vi "Framework Test.vi"(6 "max iterations":u64=1000, 10 "channel values":dbl=13579.0 format="%.4f", 11 "channel selection":T1(ring)) -> (0 "error out":errorcluster, 3 "read = write":bool)   [LabVIEW 2021, in "Reentrancy Tests.lvclass"]
uses:
  Reentrancy Tests.lvclass
  Classes/Framework/Framework.lvclass
  <vilib>/NI/Memory Manager/Classes/Pointer/Pointer.lvclass
  Classes/Configuration Session/Configuration Session.lvclass
  Classes/Configuration/Core/Framework/Framework Configuration.lvclass
  <vilib>/NI/Memory Manager/Classes/Pointer/Write DBL.vi
  <vilib>/NI/Memory Manager/Classes/Pointer/Read DBL.vi
  Typedefs/DSF Engine Framework Configuration.ctl
  DSF Core.lvlib
  Classes/Framework/Framework Options.ctl
  Typedefs/DSF Performance Options.ctl
  Typedefs/DSF FIFO Options.ctl
  Classes/Thread/Thread Options.ctl
  Classes/Thread/Thread.lvclass
  Typedefs/DSF Plugin Options.ctl
  Classes/Framework/Data Server Options.ctl
  Typedefs/DSF Settings Info.ctl
  Typedefs/DSF Engine Plugin Thread Configuration.ctl
  Typedefs/DSF Engine Channel Configuration.ctl
  Typedefs/DSF Engine Transfer Configuration.ctl
  Typedefs/DSF Engine Transfer Group Configuration.ctl
  Typedefs/DSF Engine Plugin Configuration.ctl
  Typedefs/DSF Timing Info.ctl
  Typedefs/Core Plugin Configuration.ctl
  Classes/Configuration/Core/Plugin/Plugin Configuration.lvclass
  Typedefs/Core Thread Configuration.ctl
  Classes/Configuration/Core/Thread/Thread Configuration.lvclass
  Typedefs/DSF Direction.ctl
  Typedefs/DSF Timeout Behavior.ctl
  Typedefs/Core Group Configuration.ctl
  Classes/Configuration/Core/Group/Group Configuration.lvclass
  Typedefs/Core Transfer Configuration.ctl
  Classes/Configuration/Core/Transfer/Transfer Configuration.lvclass
  Typedefs/DSF Data Type.ctl
  Typedefs/Core Channel Configuration.ctl
  Classes/Configuration/Core/Channel/Channel Configuration.lvclass
panel:
  out "iteration":u64
  in  "framework options":T2={"FIFO Options"={"Infinite Timeouts"=FALSE}, "Thread Options"={"Show FP On Call"=TRUE, "Close FP After Call"=TRUE, "Allow Debugging"=TRUE}, "Plugin Options"={"Default Components"=TRUE}, "Performance Options"={"Measure Period"=TRUE, "Measure Rx/Tx Duration"=TRUE}, "Data Server Options"={"Enable Data Server"=TRUE, "Period"=50}} {"Data Server Options"."Period" format="%d ms"}
  in  "framework configuration":T8={"plugins"=[{"core"={"name"="Plugin", "components"=[], "cycle timing"={"priority"=10000, "decimation"=1, "offset"=0}}, "component settings"=[], "threads"=[{"core"={"processor"=-2, "priority offset"=0}, "component settings"=[], "transfer groups"=[{"core"={"name"="Group", "direction"=enum."Tx", "cycle timing"={"priority"=100, "decimation"=1, "offset"=0}, "timeout behavior"=enum."Increment Late Count", "enable conversion"=FALSE}, "component settings"=[], "transfers"=[{"core"={"name"="Transfer"}, "component settings"=[], "channels"=[{"core"={"name"="Channel", "units"="V", "engine data type"=enum."DBL", "string data type"=enum."DBL", "string offset"=0}, "component settings"=[]}, {"core"={"name"="Channel", "units"="V", "engine data type"=enum."DBL", "string data type"=enum."DBL", "string offset"=0}, "component settings"=[]}, {"core"={"name"="Channel", "units"="V", "engine data type"=enum."DBL", "string data type"=enum."DBL", "string offset"=0}, "component settings"=[]}, {"core"={"name"="Channel", "units"="V", "engine data type"=enum."DBL", "string data type"=enum."DBL", "string offset"=0}, "component settings"=[]}, {"core"={"name"="Channel", "units"="V", "engine data type"=enum."DBL", "string data type"=enum."DBL", "string offset"=0}, "component settings"=[]}, {"core"={"name"="Channel", "units"="V", "engine data type"=enum."DBL", "string data type"=enum."DBL", "string offset"=0}, "component settings"=[]}, {"core"={"name"="Channel", "units"="V", "engine data type"=enum."DBL", "string data type"=enum."DBL", "string offset"=0}, "component settings"=[]}, {"core"={"name"="Channel", "units"="V", "engine data type"=enum."DBL", "string data type"=enum."DBL", "string offset"=0}, "component settings"=[]}, {"core"={"name"="Channel", "units"="V", "engine data type"=enum."DBL", "string data type"=enum."DBL", "string offset"=0}, "component settings"=[]}, {"core"={"name"="Channel", "units"="V", "engine data type"=enum."DBL", "string data type"=enum."DBL", "string offset"=0}, "component settings"=[]}, {"core"={"name"="Channel", "units"="V", "engine data type"=enum."DBL", "string data type"=enum."DBL", "string offset"=0}, "component settings"=[]}, {"core"={"name"="Channel", "units"="V", "engine data type"=enum."DBL", "string data type"=enum."DBL", "string offset"=0}, "component settings"=[]}, {"core"={"name"="Channel", "units"="V", "engine data type"=enum."DBL", "string data type"=enum."DBL", "string offset"=0}, "component settings"=[]}, {"core"={"name"="Channel", "units"="V", "engine data type"=enum."DBL", "string data type"=enum."DBL", "string offset"=0}, "component settings"=[]}, {"core"={"name"="Channel", "units"="V", "engine data type"=enum."DBL", "string data type"=enum."DBL", "string offset"=0}, "component settings"=[]}, {"core"={"name"="Channel", "units"="V", "engine data type"=enum."DBL", "string data type"=enum."DBL", "string offset"=0}, "component settings"=[]}, {"core"={"name"="Channel", "units"="V", "engine data type"=enum."DBL", "string data type"=enum."DBL", "string offset"=0}, "component settings"=[]}, {"core"={"name"="Channel", "units"="V", "engine data type"=enum."DBL", "string data type"=enum."DBL", "string offset"=0}, "component settings"=[]}, {"core"={"name"="Channel", "units"="V", "engine data type"=enum."DBL", "string data type"=enum."DBL", "string offset"=0}, "component settings"=[]}, {"core"={"name"="Channel", "units"="V", "engine data type"=enum."DBL", "string data type"=enum."DBL", "string offset"=0}, "component settings"=[]}, {"core"={"name"="Channel", "units"="V", "engine data type"=enum."DBL", "string data type"=enum."DBL", "string offset"=0}, "component settings"=[]}, {"core"={"name"="Channel", "units"="V", "engine data type"=enum."DBL", "string data type"=enum."DBL", "string offset"=0}, "component settings"=[]}, {"core"={"name"="Channel", "units"="V", "engine data type"=enum."DBL", "string data type"=enum."DBL", "string offset"=0}, "component settings"=[]}, {"core"={"name"="Channel", "units"="V", "engine data type"=enum."DBL", "string data type"=enum."DBL", "string offset"=0}, "component settings"=[]}, {"core"={"name"="Channel", "units"="V", "engine data type"=enum."DBL", "string data type"=enum."DBL", "string offset"=0}, "component settings"=[]}, {"core"={"name"="Channel", "units"="V", "engine data type"=enum."DBL", "string data type"=enum."DBL", "string offset"=0}, "component settings"=[]}, {"core"={"name"="Channel", "units"="V", "engine data type"=enum."DBL", "string data type"=enum."DBL", "string offset"=0}, "component settings"=[]}, {"core"={"name"="Channel", "units"="V", "engine data type"=enum."DBL", "string data type"=enum."DBL", "string offset"=0}, "component settings"=[]}, {"core"={"name"="Channel", "units"="V", "engine data type"=enum."DBL", "string data type"=enum."DBL", "string offset"=0}, "component settings"=[]}, {"core"={"name"="Channel", "units"="V", "engine data type"=enum."DBL", "string data type"=enum."DBL", "string offset"=0}, "component settings"=[]}, {"core"={"name"="Channel", "units"="V", "engine data type"=enum."DBL", "string data type"=enum."DBL", "string offset"=0}, "component settings"=[]}, {"core"={"name"="Channel", "units"="V", "engine data type"=enum."DBL", "string data type"=enum."DBL", "string offset"=0}, "component settings"=[]}, {"core"={"name"="Channel", "units"="V", "engine data type"=enum."DBL", "string data type"=enum."DBL", "string offset"=0}, "component settings"=[]}, {"core"={"name"="Channel", "units"="V", "engine data type"=enum."DBL", "string data type"=enum."DBL", "string offset"=0}, "component settings"=[]}, {"core"={"name"="Channel", "units"="V", "engine data type"=enum."DBL", "string data type"=enum."DBL", "string offset"=0}, "component settings"=[]}, {"core"={"name"="Channel", "units"="V", "engine data type"=enum."DBL", "string data type"=enum."DBL", "string offset"=0}, "component settings"=[]}, {"core"={"name"="Channel", "units"="V", "engine data type"=enum."DBL", "string data type"=enum."DBL", "string offset"=0}, "component settings"=[]}, {"core"={"name"="Channel", "units"="V", "engine data type"=enum."DBL", "string data type"=enum."DBL", "string offset"=0}, "component settings"=[]}, {"core"={"name"="Channel", "units"="V", "engine data type"=enum."DBL", "string data type"=enum."DBL", "string offset"=0}, "component settings"=[]}, {"core"={"name"="Channel", "units"="V", "engine data type"=enum."DBL", "string data type"=enum."DBL", "string offset"=0}, "component settings"=[]}, {"core"={"name"="Channel", "units"="V", "engine data type"=enum."DBL", "string data type"=enum."DBL", "string offset"=0}, "component settings"=[]}, {"core"={"name"="Channel", "units"="V", "engine data type"=enum."DBL", "string data type"=enum."DBL", "string offset"=0}, "component settings"=[]}, {"core"={"name"="Channel", "units"="V", "engine data type"=enum."DBL", "string data type"=enum."DBL", "string offset"=0}, "component settings"=[]}, {"core"={"name"="Channel", "units"="V", "engine data type"=enum."DBL", "string data type"=enum."DBL", "string offset"=0}, "component settings"=[]}, {"core"={"name"="Channel", "units"="V", "engine data type"=enum."DBL", "string data type"=enum."DBL", "string offset"=0}, "component settings"=[]}, {"core"={"name"="Channel", "units"="V", "engine data type"=enum."DBL", "string data type"=enum."DBL", "string offset"=0}, "component settings"=[]}, {"core"={"name"="Channel", "units"="V", "engine data type"=enum."DBL", "string data type"=enum."DBL", "string offset"=0}, "component settings"=[]}, {"core"={"name"="Channel", "units"="V", "engine data type"=enum."DBL", "string data type"=enum."DBL", "string offset"=0}, "component settings"=[]}, {"core"={"name"="Channel", "units"="V", "engine data type"=enum."DBL", "string data type"=enum."DBL", "string offset"=0}, "component settings"=[]}, {"core"={"name"="Channel", "units"="V", "engine data type"=enum."DBL", "string data type"=enum."DBL", "string offset"=0}, "component settings"=[]}, {"core"={"name"="Channel", "units"="V", "engine data type"=enum."DBL", "string data type"=enum."DBL", "string offset"=0}, "component settings"=[]}, {"core"={"name"="Channel", "units"="V", "engine data type"=enum."DBL", "string data type"=enum."DBL", "string offset"=0}, "component settings"=[]}, {"core"={"name"="Channel", "units"="V", "engine data type"=enum."DBL", "string data type"=enum."DBL", "string offset"=0}, "component settings"=[]}, {"core"={"name"="Channel", "units"="V", "engine data type"=enum."DBL", "string data type"=enum."DBL", "string offset"=0}, "component settings"=[]}, {"core"={"name"="Channel", "units"="V", "engine data type"=enum."DBL", "string data type"=enum."DBL", "string offset"=0}, "component settings"=[]}, {"core"={"name"="Channel", "units"="V", "engine data type"=enum."DBL", "string data type"=enum."DBL", "string offset"=0}, "component settings"=[]}, {"core"={"name"="Channel", "units"="V", "engine data type"=enum."DBL", "string data type"=enum."DBL", "string offset"=0}, "component settings"=[]}, {"core"={"name"="Channel", "units"="V", "engine data type"=enum."DBL", "string data type"=enum."DBL", "string offset"=0}, "component settings"=[]}, {"core"={"name"="Channel", "units"="V", "engine data type"=enum."DBL", "string data type"=enum."DBL", "string offset"=0}, "component settings"=[]}, {"core"={"name"="Channel", "units"="V", "engine data type"=enum."DBL", "string data type"=enum."DBL", "string offset"=0}, "component settings"=[]}, {"core"={"name"="Channel", "units"="V", "engine data type"=enum."DBL", "string data type"=enum."DBL", "string offset"=0}, "component settings"=[]}, {"core"={"name"="Channel", "units"="V", "engine data type"=enum."DBL", "string data type"=enum."DBL", "string offset"=0}, "component settings"=[]}, {"core"={"name"="Channel", "units"="V", "engine data type"=enum."DBL", "string data type"=enum."DBL", "string offset"=0}, "component settings"=[]}, {"core"={"name"="Channel", "units"="V", "engine data type"=enum."DBL", "string data type"=enum."DBL", "string offset"=0}, "component settings"=[]}, {"core"={"name"="Channel", "units"="V", "engine data type"=enum."DBL", "string data type"=enum."DBL", "string offset"=0}, "component settings"=[]}, {"core"={"name"="Channel", "units"="V", "engine data type"=enum."DBL", "string data type"=enum."DBL", "string offset"=0}, "component settings"=[]}, {"core"={"name"="Channel", "units"="V", "engine data type"=enum."DBL", "string data type"=enum."DBL", "string offset"=0}, "component settings"=[]}, {"core"={"name"="Channel", "units"="V", "engine data type"=enum."DBL", "string data type"=enum."DBL", "string offset"=0}, "component settings"=[]}, {"core"={"name"="Channel", "units"="V", "engine data type"=enum."DBL", "string data type"=enum."DBL", "string offset"=0}, "component settings"=[]}, {"core"={"name"="Channel", "units"="V", "engine data type"=enum."DBL", "string data type"=enum."DBL", "string offset"=0}, "component settings"=[]}, {"core"={"name"="Channel", "units"="V", "engine data type"=enum."DBL", "string data type"=enum."DBL", "string offset"=0}, "component settings"=[]}, {"core"={"name"="Channel", "units"="V", "engine data type"=enum."DBL", "string data type"=enum."DBL", "string offset"=0}, "component settings"=[]}, {"core"={"name"="Channel", "units"="V", "engine data type"=enum."DBL", "string data type"=enum."DBL", "string offset"=0}, "component settings"=[]}, {"core"={"name"="Channel", "units"="V", "engine data type"=enum."DBL", "string data type"=enum."DBL", "string offset"=0}, "component settings"=[]}, {"core"={"name"="Channel", "units"="V", "engine data type"=enum."DBL", "string data type"=enum."DBL", "string offset"=0}, "component settings"=[]}, {"core"={"name"="Channel", "units"="V", "engine data type"=enum."DBL", "string data type"=enum."DBL", "string offset"=0}, "component settings"=[]}, {"core"={"name"="Channel", "units"="V", "engine data type"=enum."DBL", "string data type"=enum."DBL", "string offset"=0}, "component settings"=[]}, {"core"={"name"="Channel", "units"="V", "engine data type"=enum."DBL", "string data type"=enum."DBL", "string offset"=0}, "component settings"=[]}, {"core"={"name"="Channel", "units"="V", "engine data type"=enum."DBL", "string data type"=enum."DBL", "string offset"=0}, "component settings"=[]}, {"core"={"name"="Channel", "units"="V", "engine data type"=enum."DBL", "string data type"=enum."DBL", "string offset"=0}, "component settings"=[]}, {"core"={"name"="Channel", "units"="V", "engine data type"=enum."DBL", "string data type"=enum."DBL", "string offset"=0}, "component settings"=[]}, {"core"={"name"="Channel", "units"="V", "engine data type"=enum."DBL", "string data type"=enum."DBL", "string offset"=0}, "component settings"=[]}, {"core"={"name"="Channel", "units"="V", "engine data type"=enum."DBL", "string data type"=enum."DBL", "string offset"=0}, "component settings"=[]}, {"core"={"name"="Channel", "units"="V", "engine data type"=enum."DBL", "string data type"=enum."DBL", "string offset"=0}, "component settings"=[]}, {"core"={"name"="Channel", "units"="V", "engine data type"=enum."DBL", "string data type"=enum."DBL", "string offset"=0}, "component settings"=[]}, {"core"={"name"="Channel", "units"="V", "engine data type"=enum."DBL", "string data type"=enum."DBL", "string offset"=0}, "component settings"=[]}, {"core"={"name"="Channel", "units"="V", "engine data type"=enum."DBL", "string data type"=enum."DBL", "string offset"=0}, "component settings"=[]}, {"core"={"name"="Channel", "units"="V", "engine data type"=enum."DBL", "string data type"=enum."DBL", "string offset"=0}, "component settings"=[]}, {"core"={"name"="Channel", "units"="V", "engine data type"=enum."DBL", "string data type"=enum."DBL", "string offset"=0}, "component settings"=[]}, {"core"={"name"="Channel", "units"="V", "engine data type"=enum."DBL", "string data type"=enum."DBL", "string offset"=0}, "component settings"=[]}, {"core"={"name"="Channel", "units"="V", "engine data type"=enum."DBL", "string data type"=enum."DBL", "string offset"=0}, "component settings"=[]}, {"core"={"name"="Channel", "units"="V", "engine data type"=enum."DBL", "string data type"=enum."DBL", "string offset"=0}, "component settings"=[]}, {"core"={"name"="Channel", "units"="V", "engine data type"=enum."DBL", "string data type"=enum."DBL", "string offset"=0}, "component settings"=[]}, {"core"={"name"="Channel", "units"="V", "engine data type"=enum."DBL", "string data type"=enum."DBL", "string offset"=0}, "component settings"=[]}, {"core"={"name"="Channel", "units"="V", "engine data type"=enum."DBL", "string data type"=enum."DBL", "string offset"=0}, "component settings"=[]}, {"core"={"name"="Channel", "units"="V", "engine data type"=enum."DBL", "string data type"=enum."DBL", "string offset"=0}, "component settings"=[]}, {"core"={"name"="Channel", "units"="V", "engine data type"=enum."DBL", "string data type"=enum."DBL", "string offset"=0}, "component settings"=[]}, {"core"={"name"="Channel", "units"="V", "engine data type"=enum."DBL", "string data type"=enum."DBL", "string offset"=0}, "component settings"=[]}, {"core"={"name"="Channel", "units"="V", "engine data type"=enum."DBL", "string data type"=enum."DBL", "string offset"=0}, "component settings"=[]}, {"core"={"name"="Channel", "units"="V", "engine data type"=enum."DBL", "string data type"=enum."DBL", "string offset"=0}, "component settings"=[]}]}]}]}]}]}
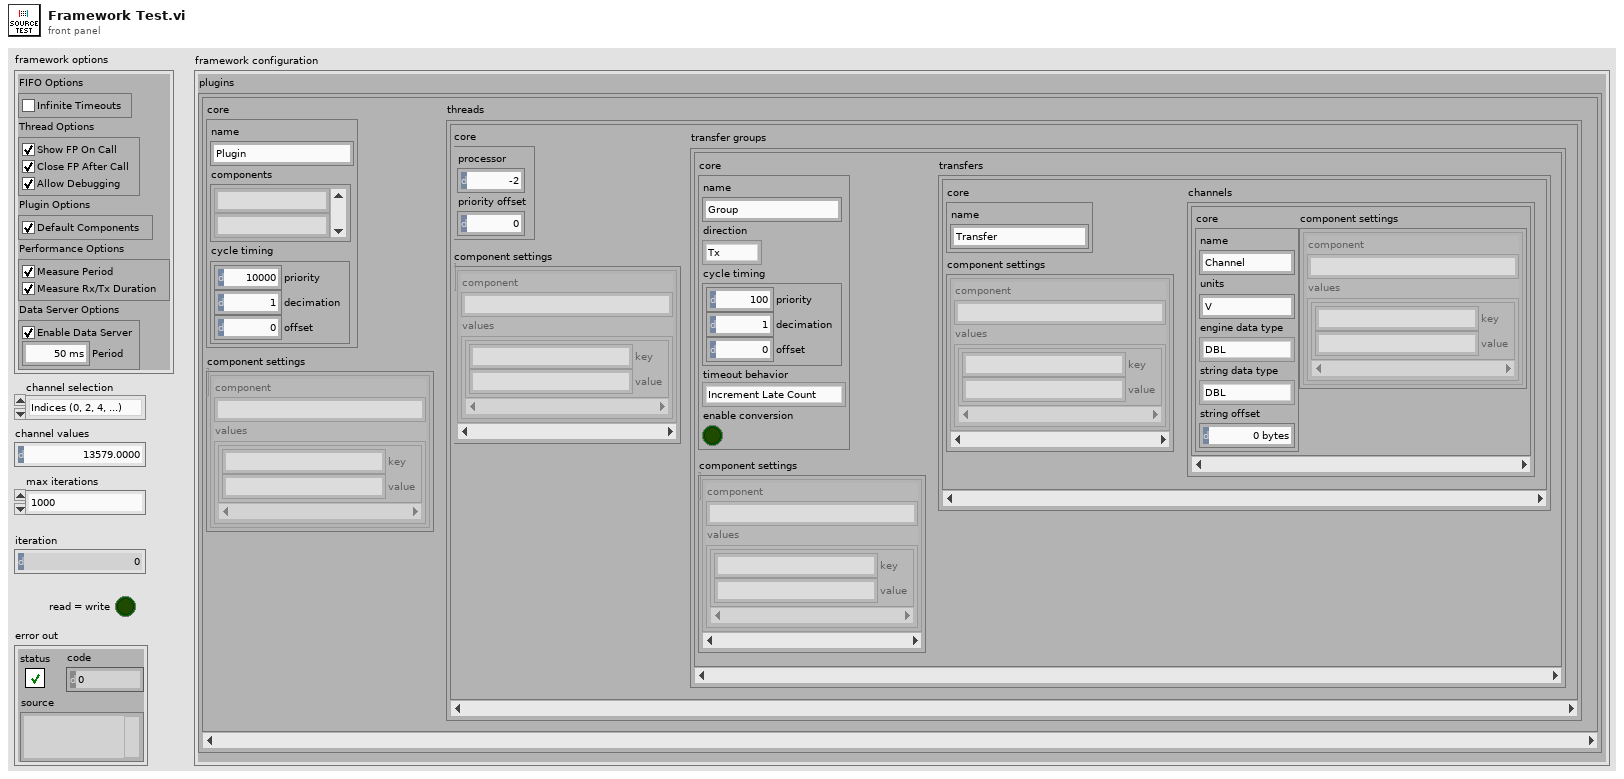
[diagram p1: front panel]
types:
  T1 = enum16{"Indices (0, 2, 4, ...)", "Indices (1, 3, 5, ...)", "All"}
  T2 = typedef "DSF Core.lvlib/Framework.lvclass/Framework Options.ctl" = cluster{"FIFO Options":T3, "Thread Options":T4, "Plugin Options":T5, "Performance Options":T6, "Data Server Options":T7}
  T3 = typedef "DSF Core.lvlib/Framework.lvclass/DSF FIFO Options.ctl" = cluster{"Infinite Timeouts":bool}
  T4 = typedef "DSF Core.lvlib/Thread.lvclass/Thread Options.ctl" = cluster{"Show FP On Call":bool, "Close FP After Call":bool, "Allow Debugging":bool}
  T5 = typedef "DSF Core.lvlib/Framework.lvclass/DSF Plugin Options.ctl" = cluster{"Default Components":bool}
  T6 = typedef "DSF Core.lvlib/DSF Performance Options.ctl" = cluster{"Measure Period":bool, "Measure Rx/Tx Duration":bool}
  T7 = typedef "DSF Core.lvlib/Framework.lvclass/Data Server Options.ctl" = cluster{"Enable Data Server":bool, "Period":u32}
  T8 = typedef "DSF Core.lvlib/DSF Engine Framework Configuration.ctl" = cluster{"plugins":T9[]}
  T9 = typedef "DSF Core.lvlib/DSF Engine Plugin Configuration.ctl" = cluster{"core":T10, "component settings":T12[], "threads":T13[]}
  T10 = typedef "DSF Core.lvlib/Plugin Configuration.lvclass/Core Plugin Configuration.ctl" = cluster{"name":string, "components":string[], "cycle timing":T11}
  T11 = typedef "DSF Core.lvlib/DSF Timing Info.ctl" = cluster{"priority":u64, "decimation":u64, "offset":u64}
  T12 = typedef "DSF Core.lvlib/DSF Settings Info.ctl" = cluster{"component":string, "values":cluster{"key":string, "value":string}[]}
  T13 = typedef "DSF Core.lvlib/DSF Engine Plugin Thread Configuration.ctl" = cluster{"core":T14, "component settings":T12[], "transfer groups":T15[]}
  T14 = typedef "DSF Core.lvlib/Thread Configuration.lvclass/Core Thread Configuration.ctl" = cluster{"processor":i32, "priority offset":i16}
  T15 = typedef "DSF Core.lvlib/DSF Engine Transfer Group Configuration.ctl" = cluster{"core":T16, "component settings":T12[], "transfers":T19[]}
  T16 = typedef "DSF Core.lvlib/Group Configuration.lvclass/Core Group Configuration.ctl" = cluster{"name":string, "direction":T17, "cycle timing":T11, "timeout behavior":T18, "enable conversion":bool}
  T17 = typedef "DSF Core.lvlib/DSF Direction.ctl" = enum8{"Tx", "Rx"}
  T18 = typedef "DSF Core.lvlib/DSF Timeout Behavior.ctl" = enum8{"Increment Late Count", "Throw Error"}
  T19 = typedef "DSF Core.lvlib/DSF Engine Transfer Configuration.ctl" = cluster{"core":T20, "component settings":T12[], "channels":T21[]}
  T20 = typedef "DSF Core.lvlib/Transfer Configuration.lvclass/Core Transfer Configuration.ctl" = cluster{"name":string}
  T21 = typedef "DSF Core.lvlib/DSF Engine Channel Configuration.ctl" = cluster{"core":T22, "component settings":T12[]}
  T22 = typedef "DSF Core.lvlib/Channel Configuration.lvclass/Core Channel Configuration.ctl" = cluster{"name":string, "units":string, "engine data type":T23, "string data type":T23, "string offset":u64}
  T23 = typedef "DSF Core.lvlib/DSF Data Type.ctl" = enum8{"Bool", "SGL", "DBL", "I8", "I16", "I32", "I64", "U8", "U16", "U32", "U64"}
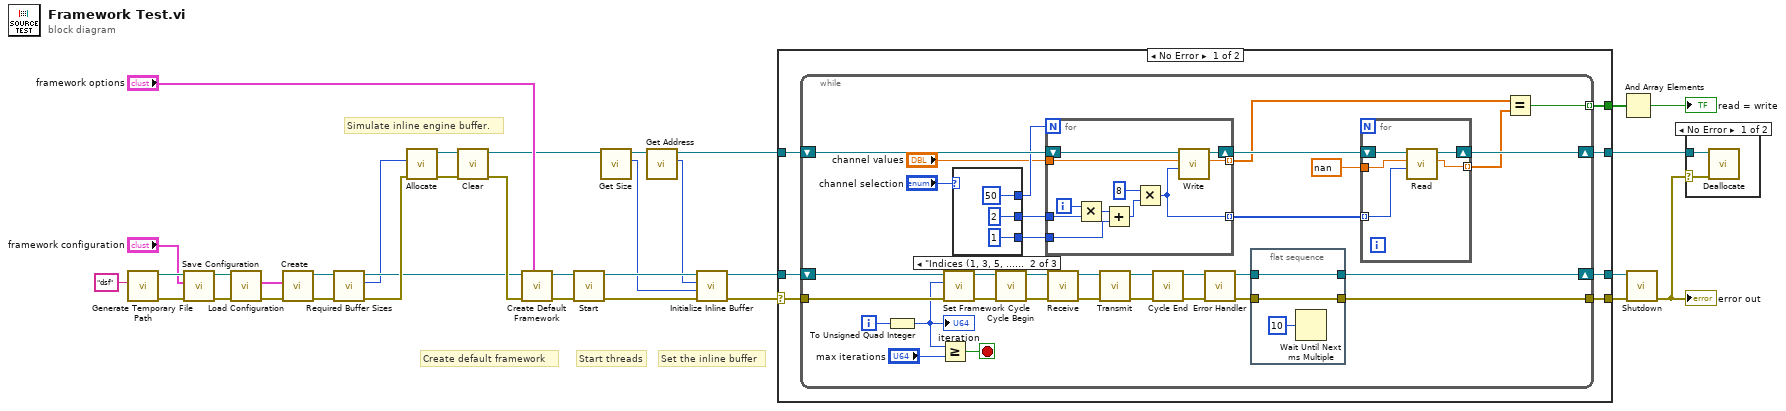
[diagram p0: block diagram]
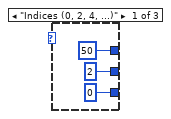
[diagram p3: hidden frame]
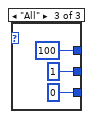
[diagram p4: hidden frame]
diagram:
  # "Set the inline buffer"
  # "Start threads"
  # "Create default framework"
  # "Simulate inline engine buffer."
  n1 = call <vilib>:"Generate Temporary File Path.vi"("Temporary File Extension (tmp)"="dsf") -> ("error out"=w17:errorcluster, "Unique Temporary File Path"=w20:path)  [unwired: 9 in]
  n2 = call "Save Configuration.vi"("error in (no error)"=w17, "framework configuration"="framework configuration", "configuration file path"=w20) -> ("error out"=w19:errorcluster, "configuration file path dup"=w18:path)  [unwired: 5 in, 2 out]
  n3 = call "Load Configuration.vi"("error in (no error)"=w19, "configuration file path"=w18) -> ("error out"=w11:errorcluster, "framework configuration"=w10:T8)  [unwired: 6 in, 2 out]
  n4 = call "Create.vi"("error in (no error)"=w11, "framework configuration"=w10) -> ("error out"=w8:errorcluster, "Framework Configuration out"=w9:refnum<class "Framework Configuration.lvclass">)  [unwired: 8 in]
  n5 = call-dynamic "Required Buffer Sizes.vi"("error in (no error)"=w8, "Framework Configuration in"=w9) -> ("error out"=w16:errorcluster, "engine size"=w13:u64, "Framework Configuration out"=w15:refnum<class "Framework Configuration.lvclass">)  [unwired: 6 in, 1 out]
  n6 = call <vilib>:"Allocate.vi"("error in (no error)"=w16, "size"=w13) -> ("error out"=w30:errorcluster, "Pointer out"=w27:refnum<class "Pointer.lvclass">)  [unwired: 8 in]
  n7 = call <vilib>:"Clear.vi"("error in (no error)"=w30, "Pointer in"=w27) -> ("error out"=w34:errorcluster, "Pointer out"=w6:refnum<class "Pointer.lvclass">)  [unwired: 8 in]
  n8 = call "Create Default Framework.vi"("framework options"="framework options", "error in (no error)"=w34, "Framework Configuration"=w15) -> ("error out"=w24:errorcluster, "Framework"=w26:refnum<class "Framework.lvclass">)  [unwired: 7 in]
  n9 = call-dynamic "Start.vi"("error in (no error)"=w24, "Framework in"=w26) -> ("error out"=w25:errorcluster, "Framework out"=w33:refnum<class "Framework.lvclass">)  [unwired: 8 in]
  n10 = call <vilib>:"Get Size.vi"("Pointer in"=w6) -> ("size"=w29:u64, "Pointer out"=w7:refnum<class "Pointer.lvclass">)  [unwired: 9 in]
  n11 = call <vilib>:"Get Address.vi"("Pointer in"=w7) -> ("address"=w28:u64, "Pointer out"=w5:refnum<class "Pointer.lvclass">)  [unwired: 9 in]
  n12 = call "Initialize Inline Buffer.vi"("error in (no error)"=w25, "size"=w29, "address"=w28, "Framework in"=w33) -> ("error out"=w23:errorcluster, "Framework out"=w22:refnum<class "Framework.lvclass">)  [unwired: 6 in]
  n13 = case shown="No Error" w23 {
    selector: w23 -> [w36 w104]
    tunnel: [w40 w104] -> w32
    tunnel: w22 -> [w38 w105]
    tunnel: [w41 w105] -> w31
    tunnel: w5 -> [w39 w103]
    tunnel: [w37 w103] -> w4
    tunnel: [w35 _] -> w1
    frame No Error {
      n14 = while {
        shift-right: [w72] -> w41
        shift-left: w38 -> [w69]
        tunnel: w36 -> [w68]
        tunnel: [w71] -> w40
        shift-right: [w48] -> w37
        shift-left: w39 -> [w57]
        tunnel: [w42] -> w35 mode=indexing
        i -> [w70]
        stop <- w53 stop-if-true
        n15 = To Unsigned Quad Integer(1:w70) -> (0:w55:u64)
        "iteration" <- w55
        n16 = Greater Or Equal?(x=w55, y="max iterations") -> (x >= y?=w53:bool)
        n17 = call "Set Framework Cycle.vi"("error in (no error)"=w68, "iteration"=w55, "Framework in"=w69) -> ("error out"=w66:errorcluster, "Framework out"=w67:refnum<class "Framework.lvclass">)  [unwired: 7 in]
        n18 = case shown="\"Indices (1, 3, 5, ...)\"" "channel selection" {
          tunnel: [50 50 100] -> w56
          tunnel: [u64 2 ("offset (0)") u64 2 ("offset (0)") u64 1 ("offset (0)")] -> w51
          tunnel: [u64 0 ("offset (0)") u64 1 ("offset (0)") u64 0 ("offset (0)")] -> w50
          frame "Indices (0, 2, 4, ...)" {
          }
          frame "Indices (1, 3, 5, ...)" {
          }
          frame "All" {
          }
        }
        n19 = call "Cycle Begin.vi"("error in (no error)"=w66, "Framework in"=w67) -> ("error out"=w64:errorcluster, "Framework out"=w65:refnum<class "Framework.lvclass">)  [unwired: 8 in]
        n20 = for {
          N: w56 -> [_]
          tunnel: "channel values" -> [w98]
          shift-right: [w96] -> w49
          shift-left: w57 -> [w99]
          tunnel: w51 -> [w94]
          tunnel: w50 -> [w92]
          tunnel: [w90] -> w47 mode=indexing
          tunnel: [w89] -> w43 mode=indexing
          i -> [w95]
          n21 = Multiply(x=w95, y=w94) -> (x*y=w93:u64)
          n22 = Add(x=w93, y=w92) -> (x+y=w91:u64)
          n23 = Multiply(x=u64 8 ("offset (0)"), y=w91) -> (x*y=w90:u64)
          n24 = call-poly <vilib>:"Write.vi"("offset (0)"=w90, "value"=w98, "Pointer in"=w99) -> ("value"=w89:dbl, "Pointer out"=w96:refnum<class "Pointer.lvclass">)  [unwired: 5 in, 2 out]
        }
        n25 = call "Receive.vi"("error in"=w64, "framework in"=w65) -> ("error out"=w74:errorcluster, "framework out"=w73:refnum<class "Framework.lvclass">)  [unwired: 8 in]
        n26 = call "Transmit.vi"("error in"=w74, "framework in"=w73) -> ("error out"=w62:errorcluster, "framework out"=w63:refnum<class "Framework.lvclass">)  [unwired: 8 in]
        n27 = call "Cycle End.vi"("error in (no error)"=w62, "Framework in"=w63) -> ("error out"=w60:errorcluster, "Framework out"=w61:refnum<class "Framework.lvclass">)  [unwired: 8 in]
        n28 = call "Error Handler.vi"("error in (no error)"=w60, "Framework in"=w61) -> ("error out"=w58:errorcluster, "Framework out"=w59:refnum<class "Framework.lvclass">)  [unwired: 8 in]
        n29 = flat-sequence {
          tunnel: w59 -> [w101]
          tunnel: w58 -> [w100]
          tunnel: [w101] -> w72
          tunnel: [w100] -> w71
          frame #0 {
            n30 = Wait Until Next ms Multiple(millisecond multiple=u32 10 ("milliseconds to wait")) -> ()  [unwired: 1 out]
          }
        }
        n31 = for {
          shift-right: [w78] -> w48
          shift-left: w49 -> [w79]
          tunnel: w47 -> [w77] mode=indexing
          tunnel: nan ("channel values") -> [w76]
          tunnel: [w75] -> w45 mode=indexing
          n32 = call-poly <vilib>:"Read.vi"("offset (0)"=w77, "value in"=w76, "Pointer in"=w79) -> ("value out"=w75:dbl, "Pointer out"=w78:refnum<class "Pointer.lvclass">)  [unwired: 5 in, 2 out]
        }
        n33 = Equal?(x=w43, y=w45) -> (x = y?=w42:bool)
      }
    }
    frame Error {
    }
  }
  n34 = And Array Elements(Boolean array=w1) -> (logical AND=→"read = write":bool)
  n35 = call-dynamic "Shutdown.vi"("error in (no error)"=w32, "Framework in"=w31) -> ("error out"=w3:errorcluster)  [unwired: 8 in, 1 out]
  "error out" <- w3
  n36 = case shown="No Error" w3 {
    selector: w3 -> [w106 _]
    tunnel: w4 -> [w107 _]
    frame No Error {
      n37 = call <vilib>:"Deallocate.vi"("error in (no error)"=w106, "Pointer"=w107) -> ()  [unwired: 8 in, 2 out]
    }
    frame Error {
    }
  }
